vi "ClimberStateMachine.vi"(9 "CimbBackButton":bool, 10 "ClimbButton":bool, 11 "State":i32) -> (0 "DisablePosCon":bool, 2 "ArmPosition":dbl, 3 "ArmForward":bool, 7 "NextState":i32)   [LabVIEW 2020]
uses:
  ClimbGlobals.vi
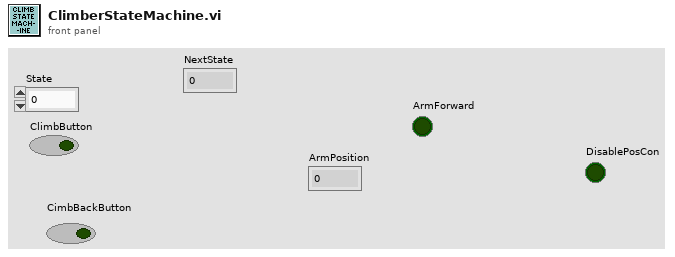
[diagram p1: front panel]
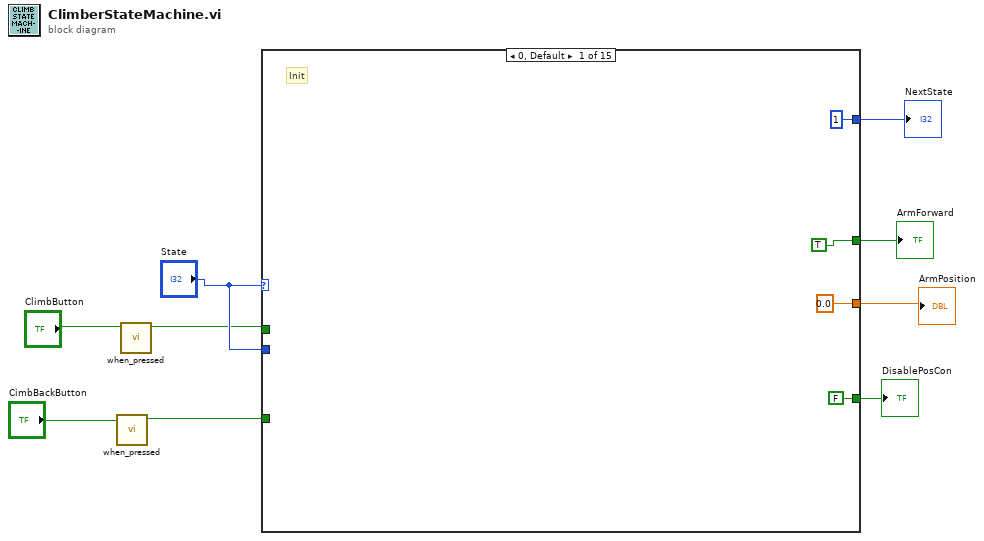
[diagram p0: block diagram]
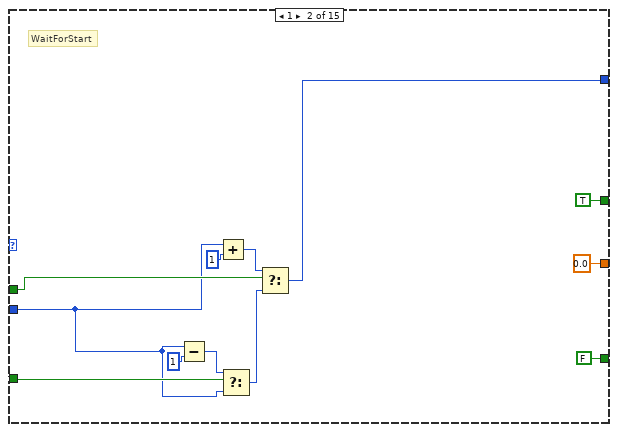
[diagram p2: hidden frame]
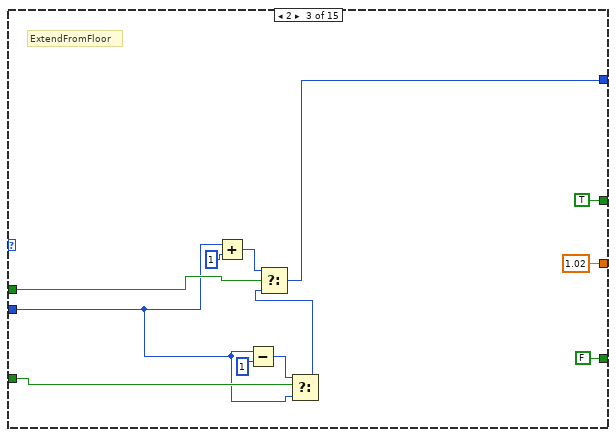
[diagram p3: hidden frame]
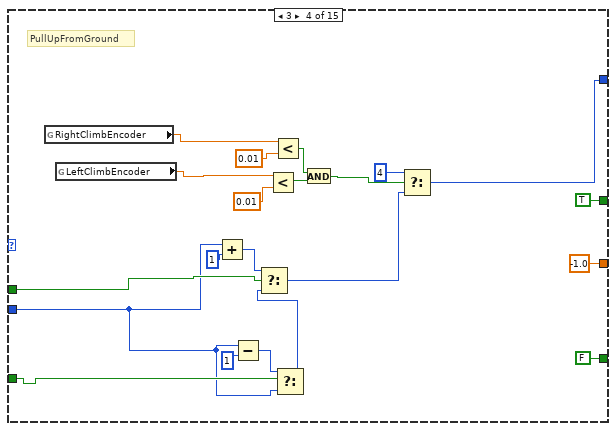
[diagram p4: hidden frame]
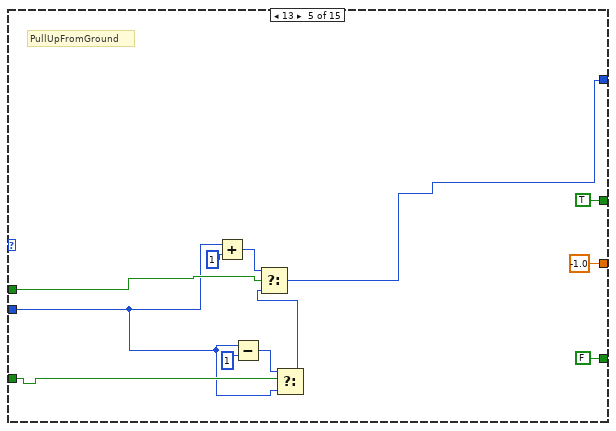
[diagram p5: hidden frame]
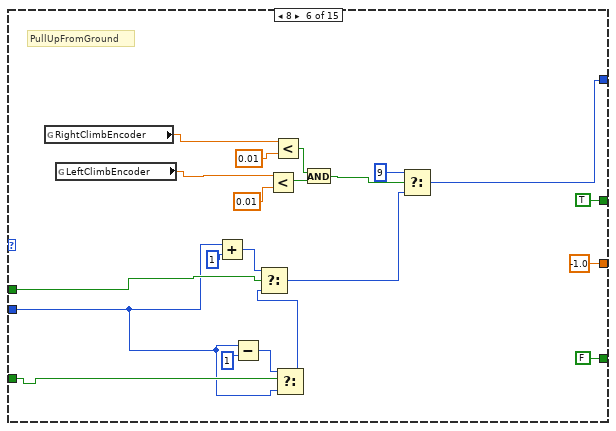
[diagram p6: hidden frame]
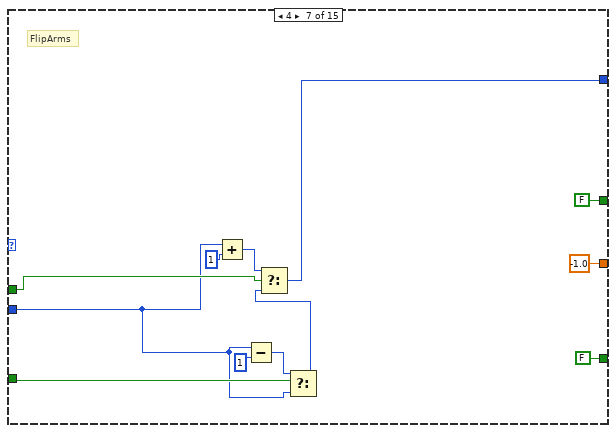
[diagram p7: hidden frame]
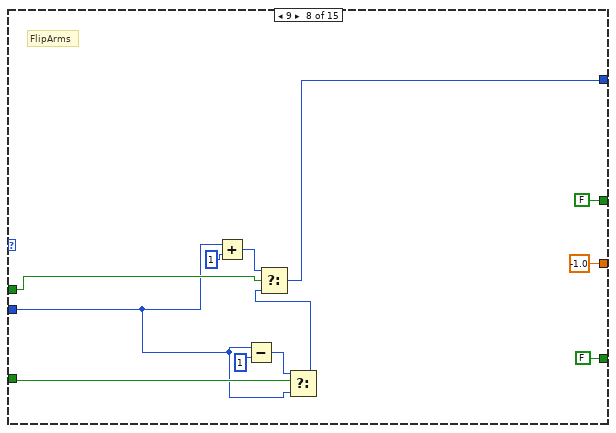
[diagram p8: hidden frame]
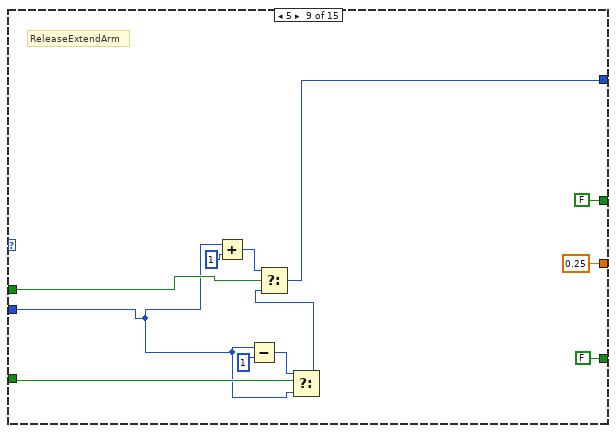
[diagram p9: hidden frame]
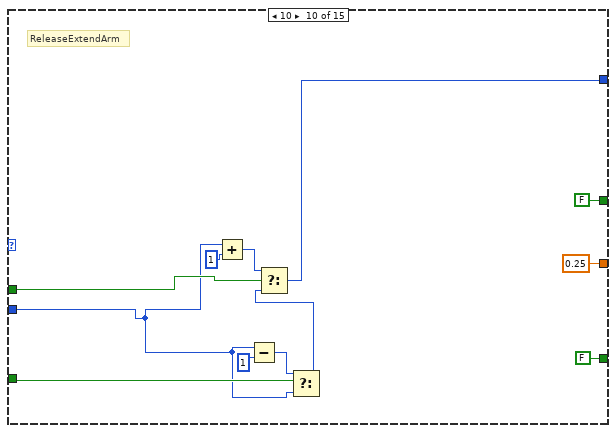
[diagram p10: hidden frame]
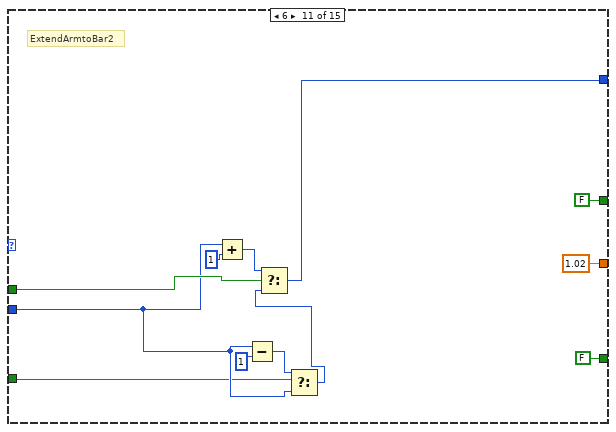
[diagram p11: hidden frame]
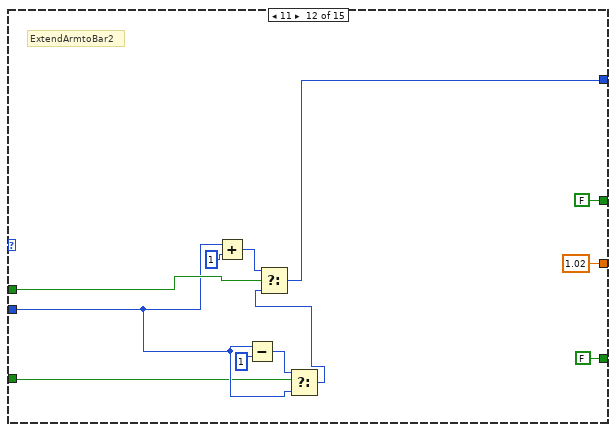
[diagram p12: hidden frame]
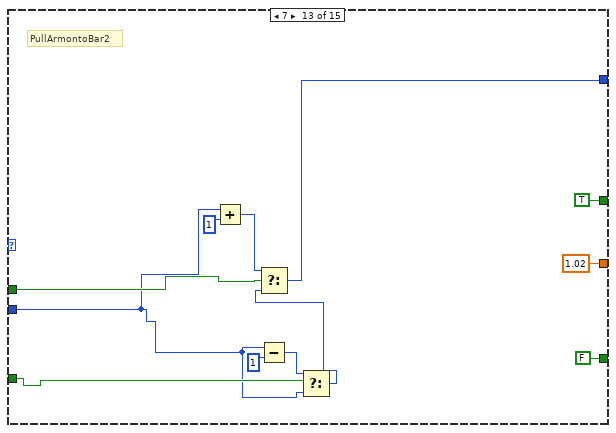
[diagram p13: hidden frame]
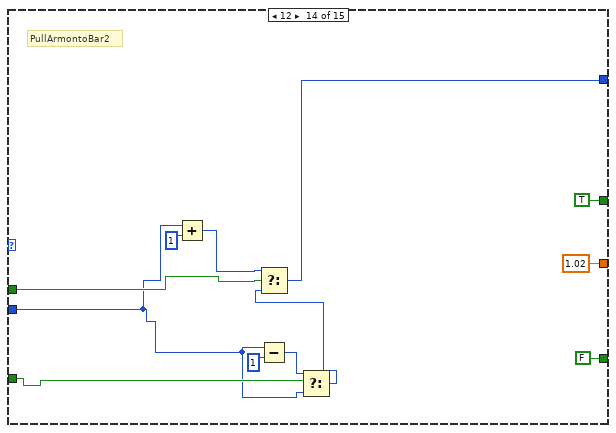
[diagram p14: hidden frame]
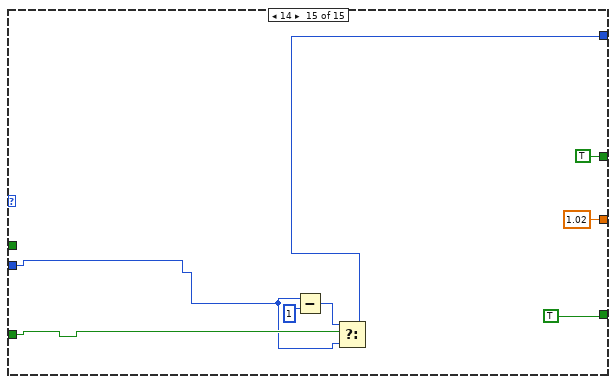
[diagram p15: hidden frame]
diagram:
  n1 = call "when_pressed.vi"("Input"="CimbBackButton") -> ("Output"=w2:bool)  [unwired: 10 in]
  n2 = call "when_pressed.vi"("Input"="ClimbButton") -> ("Output"=w5:bool)  [unwired: 10 in]
  n3 = case shown="0, Default" "State" {
    tunnel: [TRUE TRUE TRUE TRUE TRUE TRUE FALSE FALSE FALSE FALSE FALSE FALSE TRUE TRUE TRUE] -> w9
    tunnel: w5 -> [_ w20 w32 w56 w68 w89 w98 w110 w122 w134 w146 w158 w172 w184 _]
    tunnel: [1 ("State") w25 w37 w42 w59 w75 w103 w115 w127 w139 w151 w163 w175 w187 w191] -> w8
    tunnel: "State" -> [_ w16 w28 w40 w61 w74 w94 w106 w118 w130 w143 w155 w164 w176 w192]
    tunnel: [0.0 0.0 1.02 -1.0 -1.0 -1.0 -1.0 -1.0 0.25 0.25 1.02 1.02 1.02 1.02 1.02] -> w6
    tunnel: w2 -> [_ w17 w29 w48 w64 w81 w95 w107 w119 w131 w141 w153 w169 w181 w193]
    tunnel: [FALSE FALSE FALSE FALSE FALSE FALSE FALSE FALSE FALSE FALSE FALSE FALSE FALSE FALSE TRUE] -> w1
    frame 0, Default {
      # "Init"
    }
    frame 1 {
      # "WaitForStart"
      n4 = Subtract(x=w16, y=1) -> (x-y=w18:i32)
      n5 = Add(x=w16, y=1) -> (x+y=w23:i32)
      n6 = Select(t=w18, s=w17, f=w16) -> (s? t:f=w15:i32)
      n7 = Select(t=w23, s=w20, f=w15) -> (s? t:f=w25:i32)
    }
    frame 2 {
      # "ExtendFromFloor"
      n8 = Add(x=w28, y=1) -> (x+y=w35:i32)
      n9 = Subtract(x=w28, y=1) -> (x-y=w31:i32)
      n10 = Select(t=w31, s=w29, f=w28) -> (s? t:f=w27:i32)
      n11 = Select(t=w35, s=w32, f=w27) -> (s? t:f=w37:i32)
    }
    frame 3 {
      # "PullUpFromGround"
      n12 = global read "ClimbGlobals.vi" "RightClimbEncoder"() -> (w44:dbl)
      n13 = global read "ClimbGlobals.vi" "LeftClimbEncoder"() -> (w45:dbl)
      n14 = Add(x=w40, y=1) -> (x+y=w57:i32)
      n15 = Subtract(x=w40, y=1) -> (x-y=w50:i32)
      n16 = Less?(x=w45, y=0.01) -> (x < y?=w51:bool)
      n17 = Less?(x=w44, y=0.01) -> (x < y?=w52:bool)
      n18 = Select(t=w50, s=w48, f=w40) -> (s? t:f=w47:i32)
      n19 = Select(t=w57, s=w56, f=w47) -> (s? t:f=w43:i32)
      n20 = And(x=w52, y=w51) -> (x .and. y?=w39:bool)
      n21 = Select(t=4, s=w39, f=w43) -> (s? t:f=w42:i32)
    }
    frame 13 {
      # "PullUpFromGround"
      n22 = Add(x=w61, y=1) -> (x+y=w69:i32)
      n23 = Subtract(x=w61, y=1) -> (x-y=w66:i32)
      n24 = Select(t=w66, s=w64, f=w61) -> (s? t:f=w63:i32)
      n25 = Select(t=w69, s=w68, f=w63) -> (s? t:f=w59:i32)
    }
    frame 8 {
      # "PullUpFromGround"
      n26 = global read "ClimbGlobals.vi" "RightClimbEncoder"() -> (w77:dbl)
      n27 = global read "ClimbGlobals.vi" "LeftClimbEncoder"() -> (w78:dbl)
      n28 = Add(x=w74, y=1) -> (x+y=w90:i32)
      n29 = Subtract(x=w74, y=1) -> (x-y=w83:i32)
      n30 = Less?(x=w78, y=0.01) -> (x < y?=w84:bool)
      n31 = Less?(x=w77, y=0.01) -> (x < y?=w85:bool)
      n32 = Select(t=w83, s=w81, f=w74) -> (s? t:f=w80:i32)
      n33 = Select(t=w90, s=w89, f=w80) -> (s? t:f=w76:i32)
      n34 = And(x=w85, y=w84) -> (x .and. y?=w73:bool)
      n35 = Select(t=9, s=w73, f=w76) -> (s? t:f=w75:i32)
    }
    frame 4 {
      # "FlipArms"
      n36 = Add(x=w94, y=1) -> (x+y=w101:i32)
      n37 = Subtract(x=w94, y=1) -> (x-y=w97:i32)
      n38 = Select(t=w97, s=w95, f=w94) -> (s? t:f=w93:i32)
      n39 = Select(t=w101, s=w98, f=w93) -> (s? t:f=w103:i32)
    }
    frame 9 {
      # "FlipArms"
      n40 = Add(x=w106, y=1) -> (x+y=w113:i32)
      n41 = Subtract(x=w106, y=1) -> (x-y=w109:i32)
      n42 = Select(t=w109, s=w107, f=w106) -> (s? t:f=w105:i32)
      n43 = Select(t=w113, s=w110, f=w105) -> (s? t:f=w115:i32)
    }
    frame 5 {
      # "ReleaseExtendArm"
      n44 = Add(x=w118, y=1) -> (x+y=w125:i32)
      n45 = Subtract(x=w118, y=1) -> (x-y=w121:i32)
      n46 = Select(t=w121, s=w119, f=w118) -> (s? t:f=w117:i32)
      n47 = Select(t=w125, s=w122, f=w117) -> (s? t:f=w127:i32)
    }
    frame 10 {
      # "ReleaseExtendArm"
      n48 = Add(x=w130, y=1) -> (x+y=w137:i32)
      n49 = Subtract(x=w130, y=1) -> (x-y=w133:i32)
      n50 = Select(t=w133, s=w131, f=w130) -> (s? t:f=w129:i32)
      n51 = Select(t=w137, s=w134, f=w129) -> (s? t:f=w139:i32)
    }
    frame 6 {
      # "ExtendArmtoBar2"
      n52 = Add(x=w143, y=1) -> (x+y=w149:i32)
      n53 = Subtract(x=w143, y=1) -> (x-y=w145:i32)
      n54 = Select(t=w145, s=w141, f=w143) -> (s? t:f=w142:i32)
      n55 = Select(t=w149, s=w146, f=w142) -> (s? t:f=w151:i32)
    }
    frame 11 {
      # "ExtendArmtoBar2"
      n56 = Add(x=w155, y=1) -> (x+y=w161:i32)
      n57 = Subtract(x=w155, y=1) -> (x-y=w157:i32)
      n58 = Select(t=w157, s=w153, f=w155) -> (s? t:f=w154:i32)
      n59 = Select(t=w161, s=w158, f=w154) -> (s? t:f=w163:i32)
    }
    frame 7 {
      # "PullArmontoBar2"
      n60 = Add(x=w164, y=1) -> (x+y=w165:i32)
      n61 = Subtract(x=w164, y=1) -> (x-y=w171:i32)
      n62 = Select(t=w171, s=w169, f=w164) -> (s? t:f=w168:i32)
      n63 = Select(t=w165, s=w172, f=w168) -> (s? t:f=w175:i32)
    }
    frame 12 {
      # "PullArmontoBar2"
      n64 = Add(x=w176, y=1) -> (x+y=w177:i32)
      n65 = Subtract(x=w176, y=1) -> (x-y=w183:i32)
      n66 = Select(t=w183, s=w181, f=w176) -> (s? t:f=w180:i32)
      n67 = Select(t=w177, s=w184, f=w180) -> (s? t:f=w187:i32)
    }
    frame 14 {
      n68 = Subtract(x=w192, y=1) -> (x-y=w195:i32)
      n69 = Select(t=w195, s=w193, f=w192) -> (s? t:f=w191:i32)
    }
  }
  "ArmForward" <- w9
  "NextState" <- w8
  "ArmPosition" <- w6
  "DisablePosCon" <- w1
